vi "MH_TimeTag.vi"(8 "entrée d'erreur":errorcluster) -> (0 "sortie d'erreur":errorcluster, 2 "TagValue":i64, 3 "TimeTag":T1)   [LabVIEW 2019]
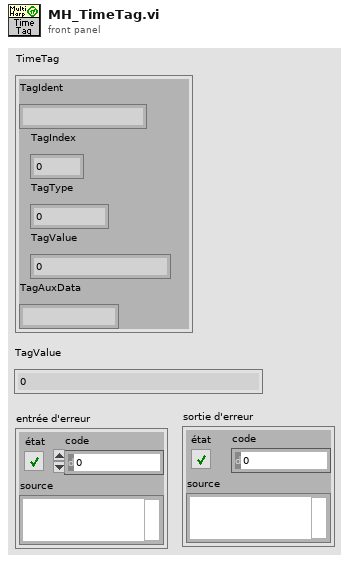
[diagram p1: front panel]
types:
  T1 = cluster{"TagIdent":string, "TagIndex":i32, "TagType":i32, "TagValue":i64, "TagAuxData":string}
  T2 = typedef "LVDateTimeRec.ctl" = cluster{"fraction de seconde":dbl, "seconde":i32, "minute":i32, "heure":i32, "jour du mois":i32, "mois":i32, "année":i32, "jour de la semaine":i32, "jour de l'année":i32, "DST":i32}
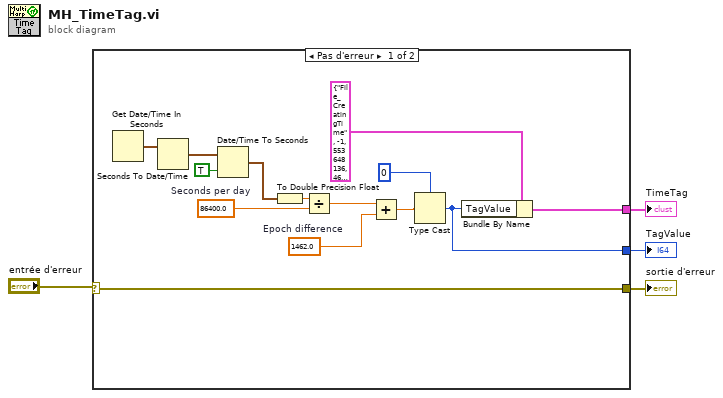
[diagram p0: block diagram]
diagram:
  n1 = case shown="Pas d'erreur" "entrée d'erreur" {
    selector: "entrée d'erreur" -> [w5 w19]
    tunnel: [w7 _] -> w4
    tunnel: [w6 _] -> w3
    tunnel: [w5 w19] -> w1
    frame No Error {
      w16 = 1462.0  # Epoch difference
      w18 = 86400.0  # Seconds per day
      n2 = Get Date/Time In Seconds() -> (seconds since 1Jan1904=w11:timestamp)
      n3 = Seconds To Date/Time(time stamp (now)=w11) -> (date time rec=w12:T2)  [unwired: 1 in]
      n4 = Date/Time To Seconds(1:TRUE ("UTC (F)"), 2:w12) -> (0:w9:timestamp)
      n5 = To Double Precision Float(number=w9) -> (double precision float=w13:dbl)
      n6 = Divide(x=w13, y=w18) -> (x/y=w17:dbl)
      n7 = Add(x=w17, y=w16) -> (x+y=w15:dbl)
      n8 = Type Cast(type=i64 0, x=w15) -> (*(type *) &x=w7:i64)
      n9 = Bundle By Name(cluster=T1 {"TagIdent"="File_CreatingTime", "TagIndex"=-1, "TagType"=553648136, "TagValue"=4676398420989345414, "TagAuxData"=""}, "TagValue"=w7) -> (w6:T1)
    }
    frame Error {
    }
  }
  "TagValue" <- w4
  "TimeTag" <- w3
  "sortie d'erreur" <- w1
